vi "Instr get_table_info.vi"(0 "table refnum":refnum<vi>) -> (1 "name_array":string[](array[string]), 2 "value_array":string[](array[string]), 3 "vaild":bool)   [LabVIEW 2018]
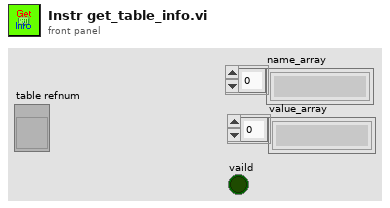
[diagram p1: front panel]
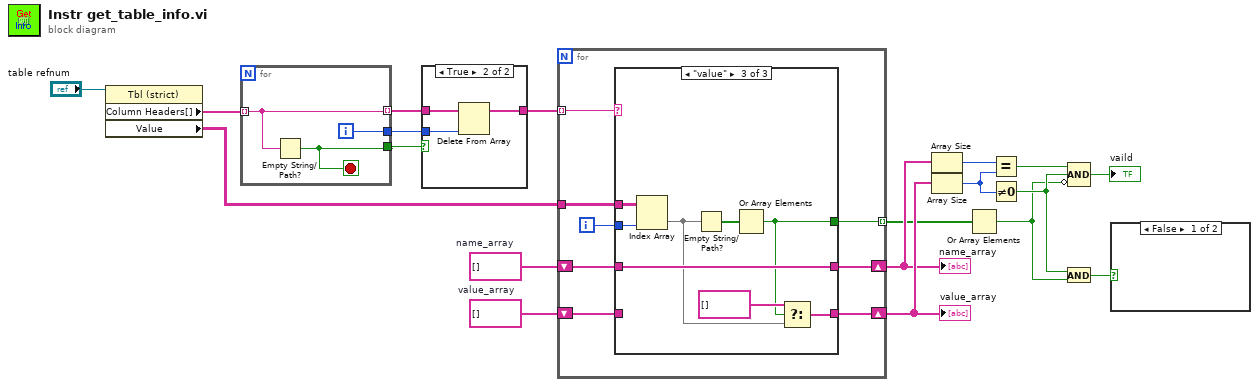
[diagram p0: block diagram]
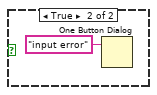
[diagram p2: hidden frame]
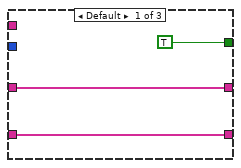
[diagram p3: hidden frame]
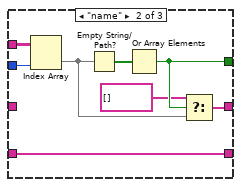
[diagram p4: hidden frame]
diagram:
  w18 = string[] []  # value_array
  w17 = string[] []  # name_array
  n1 = property class="Tbl (strict)"(reference="table refnum") -> ("Column Headers[]"=w12:string[], "Value"=w19:string[][])  [unwired: 1 in, 2 out]
  n2 = for {
    tunnel: w12 -> [w22] mode=indexing
    tunnel: [w22] -> w14 mode=indexing
    tunnel: [w21] -> w13
    tunnel: [w20] -> w15
    i -> [w20]
    stop <- w21 stop-if-true
    n3 = Empty String/Path?(string/path=w22) -> (empty?=w21:bool)
  }
  n4 = case shown="True" w13 {
    tunnel: w14 -> [w23 w26]
    tunnel: w15 -> [_ w25]
    tunnel: [w23 w24] -> w16
    frame False {
    }
    frame True {
      n5 = Delete From Array(array=w26, index=w25) -> (array with subset deleted=w24:string[])  [unwired: 1 in, 1 out]
    }
  }
  n6 = for {
    tunnel: w16 -> [w34] mode=indexing
    shift-right: [w28] -> w10
    shift-left: w17 -> [w33]
    shift-right: [w30] -> w11
    shift-left: w18 -> [w32]
    tunnel: w19 -> [w31]
    tunnel: [w27] -> w5 mode=indexing
    i -> [w29]
    n7 = case shown="\"value\"" w34 {
      tunnel: w33 -> [w37 _ w51]
      tunnel: w32 -> [w36 w45 _]
      tunnel: w31 -> [_ w44 w53]
      tunnel: [w36 w45 w47] -> w30
      tunnel: w29 -> [_ w43 w52]
      tunnel: [w37 w38 w51] -> w28
      tunnel: [TRUE w41 w46] -> w27
      frame Default {
      }
      frame "name" {
        n8 = Index Array(array=w44, index (col)=w43) -> (element=w40:string[])  [unwired: 1 in]
        n9 = Empty String/Path?(string/path=w40) -> (empty?=w42:bool[])
        n10 = Or Array Elements(Boolean array=w42) -> (logical OR=w41:bool)
        n11 = Select(t=string[] [], s=w41, f=w40) -> (s? t:f=w38:string[])
      }
      frame "value" {
        n12 = Index Array(array=w53, index (col)=w52) -> (element=w48:string[])  [unwired: 1 in]
        n13 = Empty String/Path?(string/path=w48) -> (empty?=w50:bool[])
        n14 = Or Array Elements(Boolean array=w50) -> (logical OR=w46:bool)
        n15 = Select(t=string[] [], s=w46, f=w48) -> (s? t:f=w47:string[])
      }
    }
  }
  "name_array" <- w10
  "value_array" <- w11
  n16 = Array Size(array=w10) -> (size(s)=w9:i32)
  n17 = Array Size(array=w11) -> (size(s)=w8:i32)
  n18 = Or Array Elements(Boolean array=w5) -> (logical OR=w2:bool)
  n19 = Equal?(x=w9, y=w8) -> (x = y?=w6:bool)
  n20 = Not Equal To 0?(x=w8) -> (x != 0?=w3:bool)
  n21 = And(x=w3, y=w2) -> (x .and. y?=w1:bool)
  n22 = Compound Arithmetic op=AND(w6, w3, invert w2) -> (→"vaild":bool)
  n23 = case shown="False" w1 {
    frame False {
    }
    frame True {
      n24 = One Button Dialog(message="input error") -> ()  [unwired: 1 in, 1 out]
    }
  }
